vi "Projeto.vi"() -> ()   [LabVIEW 2021]
uses:
  <vilib>/Analysis/Matrix/Datatypes/RealMatrix.ctl
  6981743f-92a7-4f7c-98ec-1d6305a85b1e.vi
  <vilib>/Array/Sort 2D Array - Pop Stack.vi
  <vilib>/Array/Sort 2D Array - Push Stack.vi
  6981743f-92a7-4f7c-98ec-1d6305a85b1e.vi/269d4b3b-47f5-49e3-8884-44851e4dd9d5.vi
  6981743f-92a7-4f7c-98ec-1d6305a85b1e.vi/6d99389c-673d-4efb-bf33-19b32bcf4cf8.vi
  <vilib>/Instr/_visa.llb/VISA Configure Serial Port (Instr).vi
  <vilib>/Analysis/Matrix/NI_Matrix.lvlib
panel:
  in  "Tab Control":enum32{"Dash", "Configurações"}(tab)
  out "Pet alimentado?":bool
  out "Numeric":dbl
  out "Porção":string
  in  "Liga/Desliga":bool
  out "Balança":u16(knob) scale=0.0..1000.0 scale format="%1d"
  in  "ADD":bool
  in  "Porta de conexão":refnum<visa-resource-name>
  in  "?":T1 {"Porção (g)" max=1000 step=10; "Minuto" max=60 step=1; "Hora" max=23 step=1}
  in  "Real Matrix":T2
  out "error out":errorcluster
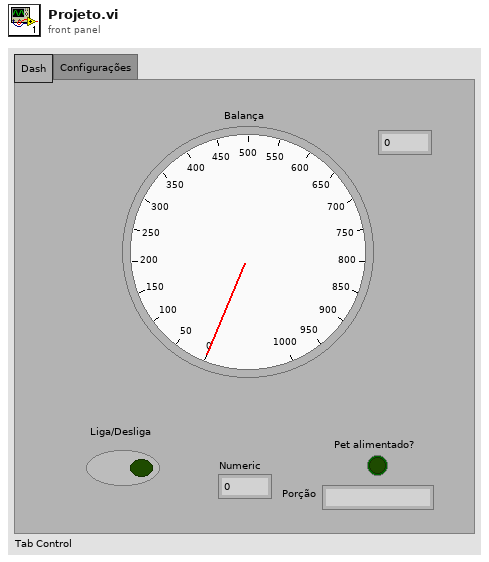
[diagram p1: front panel]
types:
  T1 = cluster{"Hora":u16, "Minuto":u16, "Porção (g)":u16}
  T2 = typedef "NI_Matrix.lvlib/RealMatrix.ctl" = dbl[][]
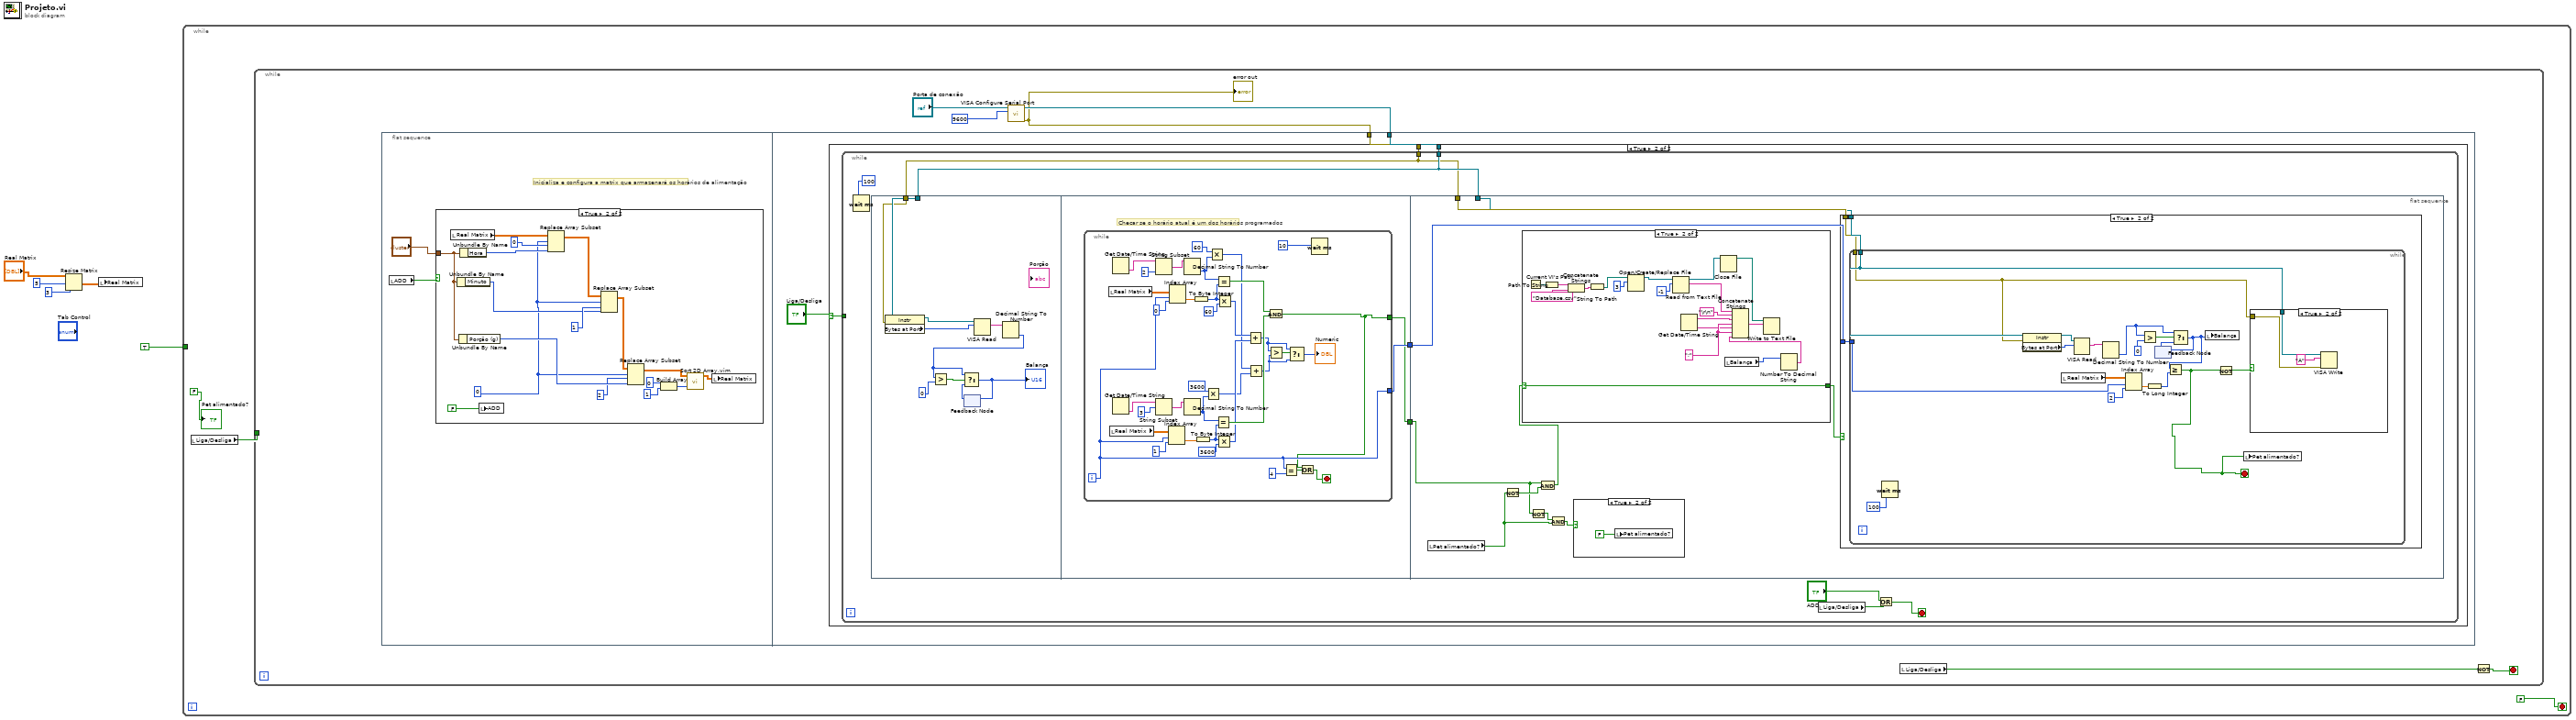
[diagram p0: block diagram]
diagram:
  n1 = Resize Matrix(1:3, 2:5, 4:"Real Matrix") -> (0:w2:T2)
  n2 = local write "Real Matrix"(w2) -> ()
  n3 = while {
    tunnel: TRUE -> [_]
    stop <- FALSE stop-if-true
    n4 = local read "Liga/Desliga"() -> (w7:bool)
    n5 = while {
      tunnel: w7 -> [_]
      stop <- w13 stop-if-true
      n6 = flat-sequence {
        tunnel: w12 -> [w36]
        tunnel: w11 -> [w35]
        frame #0 {
          # "Inicializa e configura a matrix que armazenará os horários de alimentação"
          n7 = local read "ADD"() -> (w15:bool)
          n8 = case shown="True" w15 {
            tunnel: "?" -> [_ w28]
            frame False {
            }
            frame True {
              w17 = 0
              n9 = local read "Real Matrix"() -> (w26:T2)
              n10 = Unbundle By Name(w28) -> ("Minuto"=w23:u16)
              n11 = Unbundle By Name(w28) -> ("Porção (g)"=w33:u16)
              n12 = Unbundle By Name(w28) -> ("Hora"=w32:u16)
              n13 = local write "ADD"(FALSE) -> ()
              n14 = Replace Array Subset(array=w26, new element=w32, index (row)=w17, index (col)=0) -> (w24:T2)
              n15 = Replace Array Subset(array=w24, new element=w23, index (row)=w17, index (col)=1) -> (w25:T2)
              n16 = Replace Array Subset(array=w25, new element=w33, index (row)=w17, index (col)=2) -> (w18:T2)
              n17 = Build Array(0, 1) -> (w21:i32[])
              n18 = call "Sort 2D Array.vim"("index"=w21, "2D array"=w18) -> ("sorted 2D array"=w22:dbl[][])  [unwired: 8 in, 1 out]
              n19 = local write "Real Matrix"(w22) -> ()
            }
          }
        }
        frame #1 {
          n20 = case shown="True" "Liga/Desliga" {
            selector: "Liga/Desliga" -> [_ w37]
            tunnel: w36 -> [_ w39]
            tunnel: w35 -> [_ w38]
            frame False {
            }
            frame True {
              n21 = while {
                tunnel: w39 -> [w44]
                tunnel: w38 -> [w43]
                tunnel: w37 -> [_]
                stop <- w41 stop-if-true
                n22 = Wait (ms)(milliseconds to wait=100) -> ()  [unwired: 1 out]
                n23 = flat-sequence {
                  tunnel: w44 -> [w56]
                  tunnel: w43 -> [w55]
                  tunnel: [w59] -> w47
                  tunnel: [w58] -> w46
                  tunnel: w44 -> [w104]
                  tunnel: w43 -> [w105]
                  tunnel: w47 -> [w103]
                  tunnel: w46 -> [w98]
                  frame #0 {
                    n24 = property class="Instr"(reference=w56, error in=w55) -> (reference out=w54:refnum<visa-resource-name>, "Bytes at Port"=w51:u32)  [unwired: 1 out]
                    n25 = feedback #1() -> (w48:i32)  [unwired: 1 in]
                    n26 = VISA Read(VISA resource name=w54, byte count=w51) -> (read buffer=w57:string)  [unwired: 1 in, 3 out]
                    n27 = Decimal String To Number(string=w57) -> (number=w50:i32)  [unwired: 2 in, 1 out]
                    n28 = Greater?(x=w50, y=0) -> (0:w53:bool)
                    n29 = Select(t=w50, s=w53, f=w48) -> (s? t:f=w49:i32)
                    "Balança" <- w49
                    n30 = feedback-in #1(w49) -> ()
                  }
                  frame #1 {
                    # "Checar se o horário atual é um dos horários programados"
                    n31 = while {
                      tunnel: [w61] -> w59
                      tunnel: [w60] -> w58
                      i -> [w61]
                      stop <- w78 stop-if-true
                      n32 = local read "Real Matrix"() -> (w91:T2)
                      n33 = local read "Real Matrix"() -> (w87:T2)
                      n34 = Get Date/Time String() -> (time string=w89:string)  [unwired: 3 in, 1 out]
                      n35 = Get Date/Time String() -> (time string=w94:string)  [unwired: 3 in, 1 out]
                      n36 = String Subset(string=w89, offset (0)=3) -> (substring=w90:string)  [unwired: 1 in]
                      n37 = String Subset(string=w94, length (rest)=2) -> (substring=w95:string)  [unwired: 1 in]
                      n38 = Index Array(array=w87, index (row)=w61, index (col)=1) -> (element=w80:dbl)
                      n39 = Index Array(array=w91, index (row)=w61, index (col)=0) -> (element=w81:dbl)
                      n40 = Decimal String To Number(string=w90) -> (number=w70:i32)  [unwired: 2 in, 1 out]
                      n41 = Decimal String To Number(string=w95) -> (number=w71:i32)  [unwired: 2 in, 1 out]
                      n42 = To Byte Integer(number=w81) -> (8bit integer=w75:i8)
                      n43 = To Byte Integer(number=w80) -> (8bit integer=w74:i8)
                      n44 = Multiply(x=3600, y=w70) -> (x*y=w67:i32)
                      n45 = Multiply(x=60, y=w71) -> (x*y=w66:i32)
                      n46 = Equal?(x=w70, y=w74) -> (x = y?=w84:bool)
                      n47 = Equal?(x=w71, y=w75) -> (x = y?=w85:bool)
                      n48 = Multiply(x=w74, y=3600) -> (x*y=w68:i32)
                      n49 = Multiply(x=w75, y=60) -> (x*y=w69:i32)
                      n50 = Add(x=w69, y=w68) -> (x+y=w64:i32)
                      n51 = Add(x=w66, y=w67) -> (x+y=w62:i32)
                      n52 = And(x=w85, y=w84) -> (x .and. y?=w60:bool)
                      n53 = Greater?(x=w64, y=w62) -> (0:w65:bool)
                      n54 = Equal?(x=w61, y=4) -> (x = y?=w79:bool)
                      n55 = Select(t=w64, s=w65, f=w62) -> (s? t:f=→"Numeric":i32)
                      n56 = Or(x=w60, y=w79) -> (x .or. y?=w78:bool)
                      n57 = Wait (ms)(milliseconds to wait=10) -> ()  [unwired: 1 out]
                    }
                  }
                  frame #2 {
                    n58 = local read "Pet alimentado?"() -> (w97:bool)
                    n59 = Not(x=w97) -> (.not. x?=w101:bool)
                    n60 = Not(x=w98) -> (.not. x?=w99:bool)
                    n61 = And(x=w98, y=w101) -> (x .and. y?=w100:bool)
                    n62 = case shown="True" w100 {
                      selector: w100 -> [w107 w108]
                      tunnel: [w107 w108] -> w102
                      frame False {
                      }
                      frame True {
                        w120 = ";"
                        n63 = Current VI's Path() -> (path=w124:path)
                        n64 = Path To String(path=w124) -> (string=w126:string)
                        n65 = Concatenate Strings(w126, "Database.csv") -> (w125:string)
                        n66 = String To Path(string=w125) -> (path=w114:path)
                        n67 = Open/Create/Replace File(file path (use dialog)=w114, operation (0:open)=3) -> (refnum out=w112:refnum<file>)  [unwired: 4 in, 2 out]
                        n68 = Read from Text File(file (use dialog)=w112, count=-1) -> (refnum out=w111:refnum<file>, text=w116:string)  [unwired: 2 in, 2 out]
                        n69 = Get Date/Time String() -> (date string=w118:string, time string=w119:string)  [unwired: 3 in]
                        n70 = Close File(refnum=w111) -> (path=w110:path)  [unwired: 1 in, 1 out]
                        n71 = local read "Balança"() -> (w109:u16)
                        n72 = Number To Decimal String(number=w109) -> (decimal integer string=w121:string)  [unwired: 1 in]
                        n73 = Concatenate Strings(w116, "\r\n", w118, w120, w119, w120, w121) -> (w122:string)
                        n74 = Write to Text File(file (use dialog)=w110, text=w122) -> ()  [unwired: 2 in, 3 out]
                      }
                    }
                    n75 = And(x=w99, y=w97) -> (x .and. y?=w96:bool)
                    n76 = case shown="True" w96 {
                      frame False {
                      }
                      frame True {
                        n77 = local write "Pet alimentado?"(FALSE) -> ()
                      }
                    }
                    n78 = case shown="True" w102 {
                      tunnel: w103 -> [_ w129]
                      tunnel: w104 -> [_ w128]
                      tunnel: w105 -> [_ w127]
                      frame False {
                      }
                      frame True {
                        n79 = while {
                          tunnel: w129 -> [w142]
                          tunnel: w128 -> [w140]
                          tunnel: w127 -> [w139]
                          stop <- w130 stop-if-true
                          n80 = Wait (ms)(milliseconds to wait=100) -> ()  [unwired: 1 out]
                          n81 = property class="Instr"(reference=w140, error in=w139) -> (reference out=w147:refnum<visa-resource-name>, "Bytes at Port"=w146:u32)  [unwired: 1 out]
                          n82 = local read "Real Matrix"() -> (w144:T2)
                          n83 = VISA Read(VISA resource name=w147, byte count=w146) -> (read buffer=w145:string)  [unwired: 1 in, 3 out]
                          n84 = Decimal String To Number(string=w145) -> (number=w132:i32)  [unwired: 2 in, 1 out]
                          n85 = Index Array(array=w144, index (row)=w142, index (col)=2) -> (element=w137:dbl)
                          n86 = Greater?(x=w132, y=0) -> (0:w135:bool)
                          n87 = To Long Integer(number=w137) -> (32bit integer=w138:i32)
                          n88 = feedback #2() -> (w133:i32)  [unwired: 1 in]
                          n89 = Select(t=w132, s=w135, f=w133) -> (s? t:f=w131:i32)
                          n90 = feedback-in #2(w131) -> ()
                          n91 = Greater Or Equal?(x=w131, y=w138) -> (x >= y?=w130:bool)
                          n92 = local write "Balança"(w131) -> ()
                          n93 = Not(x=w130) -> (.not. x?=w141:bool)
                          n94 = local write "Pet alimentado?"(w130) -> ()
                          n95 = case shown="True" w141 {
                            tunnel: w140 -> [_ w150]
                            tunnel: w139 -> [_ w149]
                            frame False {
                            }
                            frame True {
                              n96 = VISA Write(VISA resource name=w150, write buffer="A", error in (no error)=w149) -> ()  [unwired: 3 out]
                            }
                          }
                        }
                      }
                    }
                  }
                }
                n97 = local read "Liga/Desliga"() -> (w42:bool)
                n98 = Or(x="ADD", y=w42) -> (x .or. y?=w41:bool)
              }
            }
          }
        }
      }
      n99 = call-poly "VISA Configure Serial Port"("VISA resource name"="Porta de conexão", "baud rate (9600)"=u32 9600) -> ("VISA resource name out"=w12:refnum<visa-resource-name>, "error out"=w11:errorcluster)  [unwired: 12 in]
      "error out" <- w11
      n100 = local read "Liga/Desliga"() -> (w14:bool)
      n101 = Not(x=w14) -> (.not. x?=w13:bool)
    }
    "Pet alimentado?" <- FALSE
  }
